vi "Yokogawa - set mode.vi"(8 "error in (no error)":errorcluster, 10 "Mode (0: Normal)":u16(ring) items=["Normal", "Harmonics"], 11 "VISA Refnum in":refnum<visa-resource-name>) -> (0 "error out":errorcluster, 3 "VISA Refnum out":refnum<visa-resource-name>)   [LabVIEW 2013]
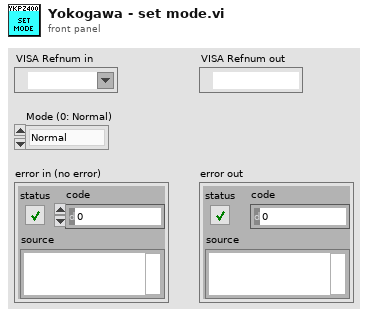
[diagram p1: front panel]
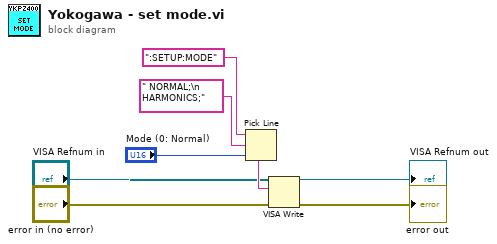
[diagram p0: block diagram]
diagram:
  n1 = Pick Line(string ("")=":SETUP:MODE", multi-line string=" NORMAL;\n HARMONICS;", line index="Mode (0: Normal)") -> (output string=w8:string)
  n2 = VISA Write(VISA resource name="VISA Refnum in", write buffer=w8, error in (no error)="error in (no error)") -> (VISA resource name out=→"VISA Refnum out":refnum<visa-resource-name>, error out=→"error out":errorcluster)  [unwired: 1 out]
